vi "RT to GUI Step.vi"(0 "STEP":T1={"Direction"=enum."Chamber", "Pressure MPa"=0.0, "Time s"=0.0, "Delta alarm MPa"=0.0, "Delta warning MPa"=0.0}) -> (4 "GUI Step":T3)   [LabVIEW 2019]
uses:
  TypeDef/GUI Step.ctl
  TypeDef/Step.ctl
  TypeDef/Direction.ctl
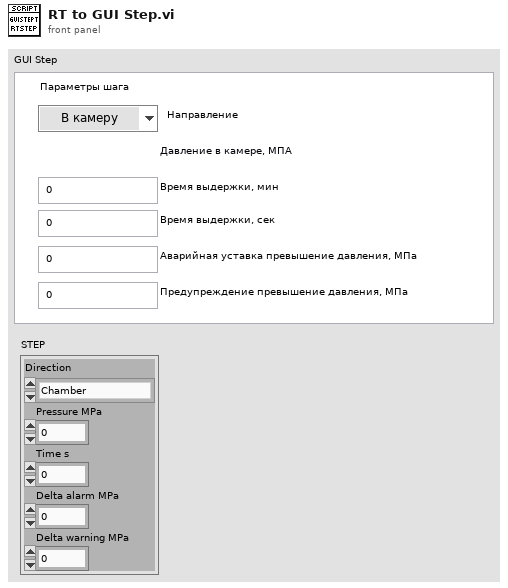
[diagram p1: front panel]
types:
  T1 = typedef "Step.ctl" = cluster{"Direction":T2, "Pressure MPa":dbl, "Time s":dbl, "Delta alarm MPa":dbl, "Delta warning MPa":dbl}
  T2 = typedef "Direction.ctl" = enum16{"None", "Chamber", "DUT"}
  T3 = typedef "GUI Step.ctl" = cluster{"pressure MPa":dbl, "time min":dbl, "delta alarm MPa":dbl, "direction":enum16{"В камеру", "В образец"}, "delta warning MPa":dbl, "time sec":dbl}
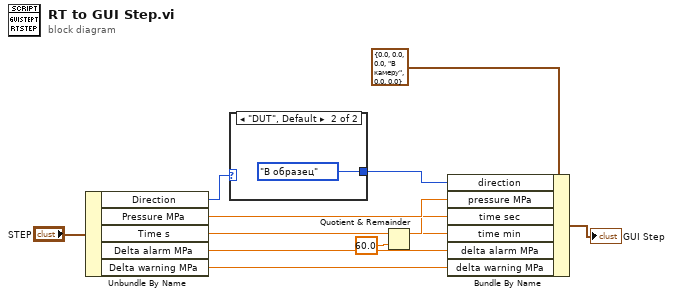
[diagram p0: block diagram]
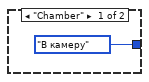
[diagram p2: hidden frame]
diagram:
  n1 = Unbundle By Name("STEP") -> ("Direction"=w12:T2, "Pressure MPa"=w7:dbl, "Time s"=w6:dbl, "Delta alarm MPa"=w2:dbl, "Delta warning MPa"=w1:dbl)
  n2 = case shown="\"DUT\", Default" w12 {
    tunnel: [enum16{"В камеру", "В образец"}."В камеру" ("direction") enum16{"В камеру", "В образец"}."В образец" ("direction")] -> w8
    frame "Chamber" {
    }
    frame "DUT", Default {
    }
  }
  n3 = Quotient & Remainder(x=w6, y=60.0) -> (x-y*floor(x/y)=w4:dbl, floor(x/y)=w3:dbl)
  n4 = Bundle By Name(cluster=T3 {"pressure MPa"=0.0, "time min"=0.0, "delta alarm MPa"=0.0, "direction"=enum."В камеру", "delta warning MPa"=0.0, "time sec"=0.0} ("GUI Step"), "direction"=w8, "pressure MPa"=w7, "time sec"=w4, "time min"=w3, "delta alarm MPa"=w2, "delta warning MPa"=w1) -> (→"GUI Step":T3)
